vi "Config Loaded from DB.vi"(8 "error in":errorcluster, 11 "Sim Signal Config":T1={"offset"=0.0, "square wave duty cycle (%)"=50.0, "signal type"=enum."Sine Wave", "phase"=0.0, "amplitude"=1.0, "frequency"=10.0, "sampling info"={"Fs"=1000.0, "#s"=1000.0}} {"sampling info"."Fs" format="%.2p"; "frequency" scale=0.0..10.0; "amplitude" scale=0.0..10.0; "phase" format="%.2p"; "square wave duty cycle (%)" format="%0.2f"; "offset" scale=0.0..10.0}) -> (0 "error out":errorcluster)   [LabVIEW 2020, in "Config.lvlib"]
doc: "Config Loaded froma Data Base\n_____\nCreated using Delacor QMH Event Scripter 6.0.0.121."
uses:
  Config.lvlib
  sim signal -- cluster.ctl
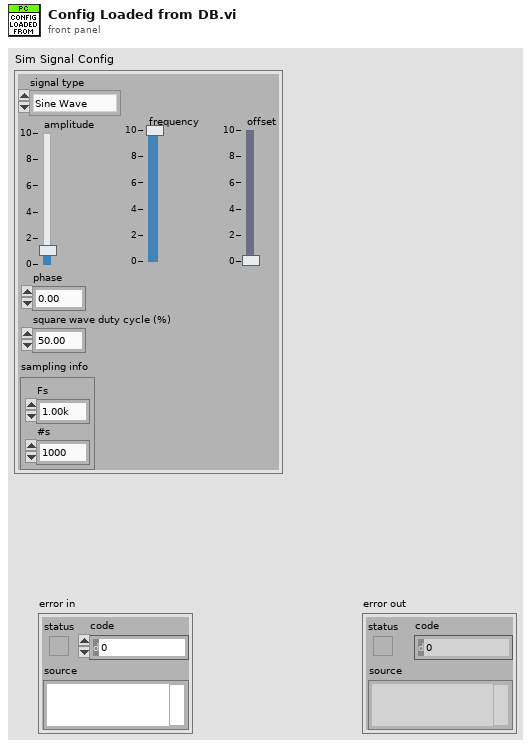
[diagram p1: front panel]
types:
  T1 = typedef "Config.lvlib/sim signal -- cluster.ctl" = cluster{"offset":dbl, "square wave duty cycle (%)":dbl, "signal type":enum16{"Sine Wave", "Triangle Wave", "Square Wave", "Sawtooth Wave"}, "phase":dbl, "amplitude":dbl, "frequency":dbl, "sampling info":cluster{"Fs":dbl, "#s":dbl}}
  T2 = typedef "Config.lvlib/Request Events--cluster.ctl" = cluster{"Stop Module":refnum<user-event>, "Show Panel":refnum<user-event>, "Hide Panel":refnum<user-event>, "Get Module Execution Status":refnum<user-event>, "Show Diagram":refnum<user-event>, "Save Config":refnum<user-event>, "Cancel config":refnum<user-event>, "Load Config":refnum<user-event>, "Config Loaded from DB":refnum<user-event>}
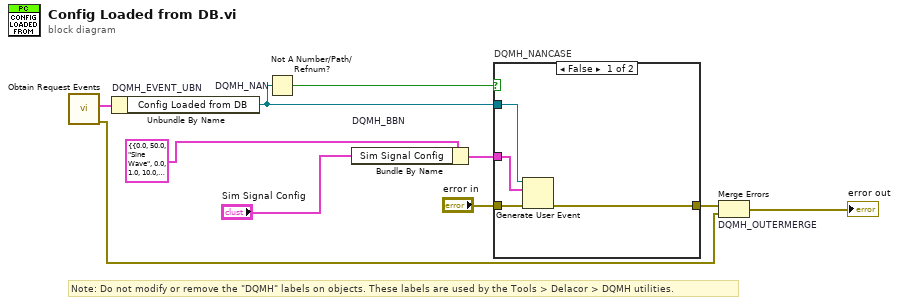
[diagram p0: block diagram]
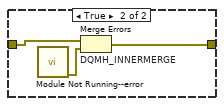
[diagram p2: hidden frame]
diagram:
  # "Note: Do not modify or remove the \"DQMH\" labels on objects. These labels are used by the Tools > Delacor > DQMH utilities."
  n1 = call "Obtain Request Events.vi"() -> ("error out"=w4:errorcluster, "Config Request Events"=w3:T2)  [unwired: 10 in]
  n2 = Unbundle By Name "DQMH_EVENT_UBN"(w3) -> ("Config Loaded from DB"=w6:refnum<user-event>)
  n3 = Not A Number/Path/Refnum? "DQMH_NAN"(number/path/refnum=w6) -> (NaN/Path/Refnum?=w7:bool)
  n4 = Bundle By Name "DQMH_BBN"(cluster=cluster{"Sim Signal Config":T1} {"Sim Signal Config"={"offset"=0.0, "square wave duty cycle (%)"=50.0, "signal type"=enum."Sine Wave", "phase"=0.0, "amplitude"=1.0, "frequency"=10.0, "sampling info"={"Fs"=1000.0, "#s"=1000.0}}} ("Cluster"), "Sim Signal Config"="Sim Signal Config") -> (w8:cluster{"Sim Signal Config":T1})
  n5 = case "DQMH_NANCASE" shown="False" w7 {
    tunnel: "error in" -> [w14 w17]
    tunnel: [w13 w16] -> w5
    tunnel: w6 -> [w12 _]
    tunnel: w8 -> [w11 _]
    frame False {
      n6 = Generate User Event(user event=w12, event data cluster=w11, error in=w14) -> (error out=w13:errorcluster)  [unwired: 1 in, 1 out]
    }
    frame True {
      n7 = call "Module Not Running--error.vi"() -> ("error out"=w15:errorcluster)  [unwired: 11 in]
      n8 = Merge Errors "DQMH_INNERMERGE"(w17, w15) -> (w16:errorcluster)
    }
  }
  n9 = Merge Errors "DQMH_OUTERMERGE"(w5, w4) -> (→"error out":errorcluster)
